vi "temp chart with pid.vi"(0 "Slave Controls":bool, 1 "exit T control":bool, 7 "Control Parameters":T4={"Setpoint"=50.0, "Control bandwidth"=4.0, "Settle bandwidth"=1.0, "Integral time"=30.0, "Int\non"=TRUE, "Derivative time"=0.5, "Der\non"=TRUE, "Settle time"=60.0} {"Settle time" format="%.2f"; "Derivative time" format="%.2f"; "Integral time" format="%.2f"; "Settle bandwidth" format="%.2f"; "Control bandwidth" format="%.2f"; "Setpoint" format="%.2f"}, 11 "error in":errorcluster, 12 "Manual Override":bool) -> (8 "Temp":dbl format="%.2f", 10 "Time in Settle Band":dbl format="%.2f", 14 "settled":bool, 15 "error out":errorcluster)   [LabVIEW 2016]
doc: "This vi records and plots the temperature of a 10 kOhm thermsitor using an Agilent 34405A as the measurment device.\n\nIt sets the power to the heater resistor using the NI ELVIS Variable DC, and measures the power using DAQ analog in.\n\nIt uses a PID feedback algorithm to obtain the desired setpoint.\n\nPaul K Dixon\nPhysics 350\nCSUSB Physics"
uses:
  typedefs/control parameters.ctl
  typedefs/status indicator.ctl
  typedefs/scale control.ctl
  <vilib>/Utility/miscctls.llb/LVPointTypeDef.ctl
  globals/temp control global variables.vi
panel:
  in  "Slave Scale":bool=TRUE
  out "Logging":bool
  in  "Scale Control":T1
  in  "Power Control":dbl(slide) scale=0.0..1.0
  out "range indicators":T2={"In control band"=FALSE, "In settle band"=FALSE, "under range"=TRUE, "over range"=FALSE}
  out "Power":dbl=0.754407202908737 format="%.2f"
  out "Setpoint":dbl=50.0 format="%.2f"
  in  "shrink":bool
  in  "expand":bool
  out "Temperature History":T3(graph)={"temp out"=29.702811899974034, 50.0, 50.5, 49.5, 50.1, 49.9, 50.508814405817475}
  # "PID Temperature Controller"
  # "1.0"
  # "Norm\nPower\nscale"
  # "0.5"
  # "0.0"
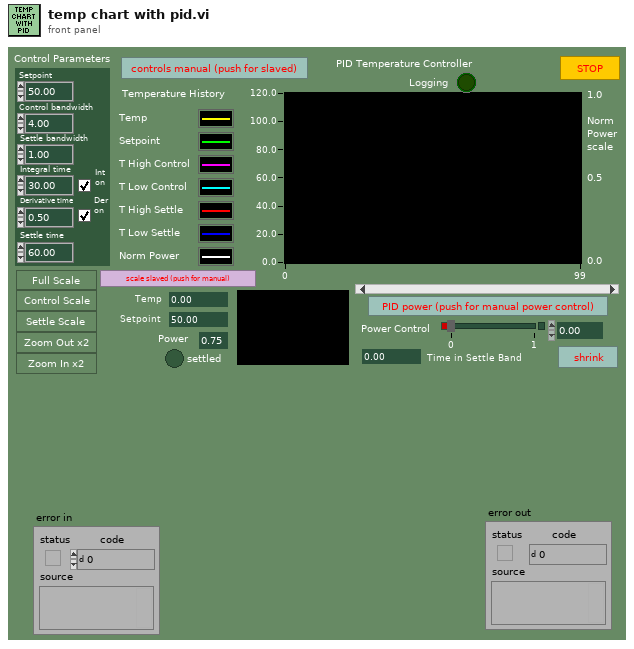
[diagram p1: front panel]
types:
  T1 = typedef "scale control.ctl" = cluster{"Full Scale":bool, "Control Scale":bool, "Settle Scale":bool, "Zoom Out":bool, "Zoom In":bool}
  T2 = typedef "status indicator.ctl" = cluster{"In control band":bool, "In settle band":bool, "under range":bool, "over range":bool}
  T3 = cluster{"temp out":dbl, dbl, dbl, dbl, dbl, dbl, dbl}
  T4 = typedef "control parameters.ctl" = cluster{"Setpoint":dbl, "Control bandwidth":dbl, "Settle bandwidth":dbl, "Integral time":dbl, "Int\non":bool, "Derivative time":dbl, "Der\non":bool, "Settle time":dbl}
  T5 = typedef "LVPointTypeDef.ctl" = cluster{"Horizontal":i16, "Vertical":i16}
  T6 = cluster{"[0]":refnum<vi>, "[1]":refnum<vi>, "[2]":refnum<vi>, "[3]":refnum<vi>}
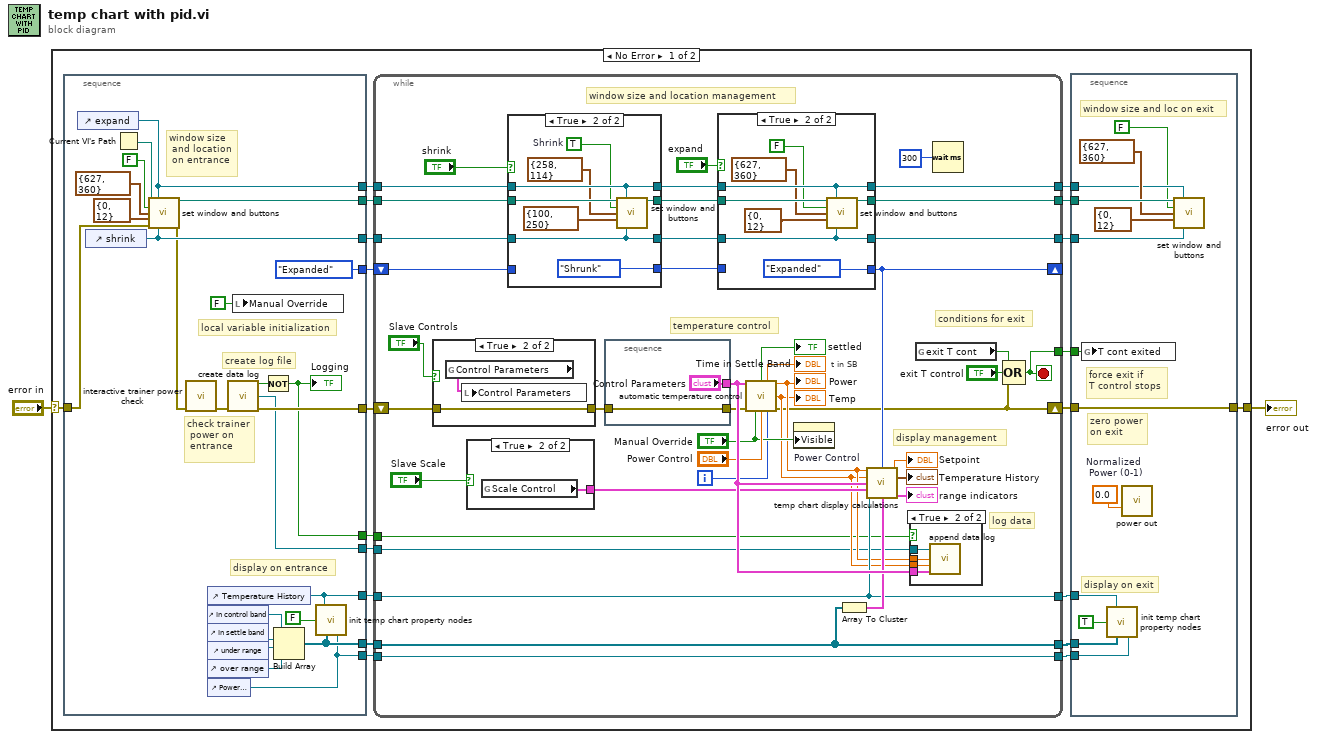
[diagram p0: block diagram]
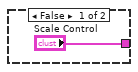
[diagram p2: hidden frame]
diagram:
  n1 = case shown="No Error" "error in" {
    selector: "error in" -> [w20 w137]
    tunnel: [w21 w137] -> w1
    frame No Error {
      n2 = stacked-sequence {
        tunnel: w20 -> [w128]
        tunnel: [w135] -> w19
        tunnel: [w130] -> w17
        tunnel: [w129] -> w16
        tunnel: [w125] -> w12
        tunnel: [w126] -> w11
        tunnel: [w123] -> w7
        tunnel: [w121] -> w6
        tunnel: [w118] -> w5
        tunnel: [w117] -> w4
        tunnel: [enum16{"Expanded", "Shrunk"}."Expanded" ("Mode")] -> w3
        frame #0 {
          # "create log file"
          # "local variable initialization"
          # "display on entrance"
          # "check trainer\n power on\n entrance"
          # "window size\n and location\n on entrance"
          n3 = control-ref of="expand"() -> (w130:refnum<vi>)
          n4 = control-ref of="shrink"() -> (w129:refnum<vi>)
          n5 = Current VI's Path() -> (path=w136:path)
          n6 = call "set window and buttons.vi"("path in"=w136, "expand ref"=w130, "Shrink"=FALSE, "Window Dimensions"=cluster{"window width":i16, "window height":i16} {"window width"=627, "window height"=360} ("Default LTWH"), "Origin"=T5 {"Horizontal"=0, "Vertical"=12}, "error in"=w128, "shrink ref"=w129) -> ("path out"=w135:path, "error out"=w127:errorcluster)  [unwired: 7 out]
          n7 = call "interactive trainer power check.vi"("error in"=w127) -> ("error out"=w122:errorcluster)  [unwired: 14 out]
          n8 = control-ref of="Temperature History"() -> (w126:refnum<vi>)
          n9 = control-ref of="In control band"() -> (w131:refnum<vi>)
          n10 = control-ref of="In settle band"() -> (w132:refnum<vi>)
          n11 = control-ref of="under range"() -> (w133:refnum<vi>)
          n12 = control-ref of="over range"() -> (w134:refnum<vi>)
          n13 = control-ref of="Power Control"() -> (w123:refnum<vi>)
          n14 = call "create data log.vi"("error in"=w122) -> ("cancelled"=w119:bool, "file refnum out"=w118:refnum<file>, "error out"=w121:errorcluster)  [unwired: 1 in, 11 out]
          n15 = local write "Manual Override"(FALSE ("Manual Override")) -> ()
          n16 = Not(x=w119) -> (.not. x?=w117:bool)
          "Logging" <- w117
          n17 = Build Array(w131, w132, w133, w134) -> (w125:refnum<vi>[])
          n18 = call "init temp chart property nodes.vi"("Temperature History"=w126, "Power control visible"=FALSE ("Visible"), "range indicators"=w125, "Power Control"=w123) -> ()  [unwired: 2 in, 10 out]
        }
      }
      n19 = while {
        tunnel: w7 -> [w37]
        tunnel: [w37] -> w8
        tunnel: [w38] -> w9
        tunnel: [w39] -> w10
        tunnel: w11 -> [w38]
        tunnel: w12 -> [w39]
        tunnel: [w41] -> w13
        tunnel: [w42] -> w14
        tunnel: [w43] -> w15
        tunnel: w16 -> [w48]
        tunnel: w17 -> [w49]
        tunnel: [w51] -> w18
        tunnel: w19 -> [w62]
        shift-left: w6 -> [w26]
        shift-right: [w27] -> w22
        tunnel: w5 -> [w32]
        tunnel: w4 -> [w31]
        shift-right: [w28] -> _
        shift-left: w3 -> [w30]
        i -> [w35]
        stop <- w51 stop-if-true
        # "log data"
        # "display management"
        # "conditions for exit"
        # "temperature control"
        # "t in SB"
        # "window size and location management"
        n20 = case shown="True" "Slave Controls" {
          tunnel: w26 -> [w67 w68]
          tunnel: [w67 w68] -> w25
          frame False {
          }
          frame True {
            n21 = global read "temp control global variables.vi" "Control Parameters"() -> (w69:T4)
            n22 = local write "Control Parameters"(w69) -> ()
          }
        }
        n23 = case shown="True" "Slave Scale" {
          tunnel: ["Scale Control" w66] -> w53
          frame False {
          }
          frame True {
            n24 = global read "temp control global variables.vi" "Scale Control"() -> (w66:T1)
          }
        }
        n25 = case shown="True" "shrink" {
          tunnel: w62 -> [w91 w99]
          tunnel: [w91 w98] -> w46
          tunnel: w49 -> [w90 w97]
          tunnel: w48 -> [w89 w96]
          tunnel: [w90 w97] -> w45
          tunnel: [w89 w96] -> w44
          tunnel: w30 -> [w88 _]
          tunnel: [w88 enum16{"Expanded", "Shrunk"}."Shrunk" ("Mode")] -> w29
          frame False {
          }
          frame True {
            w94 = TRUE  # Shrink
            n26 = call "set window and buttons.vi"("path in"=w99, "expand ref"=w97, "Shrink"=w94, "Window Dimensions"=cluster{"window width":i16, "window height":i16} {"window width"=258, "window height"=114} ("Default LTWH"), "Origin"=T5 {"Horizontal"=100, "Vertical"=250}, "shrink ref"=w96) -> ("path out"=w98:path)  [unwired: 1 in, 8 out]
          }
        }
        n27 = stacked-sequence {
          tunnel: ["Control Parameters"] -> w64
          tunnel: w25 -> [w86]
          tunnel: [w86] -> w50
          frame #0 {
          }
        }
        n28 = case shown="True" "expand" {
          tunnel: w46 -> [w77 w85]
          tunnel: [w77 w84] -> w43
          tunnel: w45 -> [w76 w83]
          tunnel: w44 -> [w75 w82]
          tunnel: [w76 w83] -> w41
          tunnel: [w75 w82] -> w42
          tunnel: w29 -> [w74 _]
          tunnel: [w74 enum16{"Expanded", "Shrunk"}."Expanded" ("Mode")] -> w28
          frame False {
          }
          frame True {
            n29 = call "set window and buttons.vi"("path in"=w85, "expand ref"=w83, "Shrink"=FALSE, "Window Dimensions"=cluster{"window width":i16, "window height":i16} {"window width"=627, "window height"=360} ("Default LTWH"), "Origin"=T5 {"Horizontal"=0, "Vertical"=12}, "shrink ref"=w82) -> ("path out"=w84:path)  [unwired: 1 in, 8 out]
          }
        }
        n30 = call "automatic temperature control.vi"("Control Parameters"=w64, "error in"=w50, "Manual Override"="Manual Override", "Normalized Power In (0-1)"="Power Control", "index (0=init)"=w35) -> ("settled"=→"settled":bool, "time in settle band"=→"Time in Settle Band":dbl, "power meas (0-1)"=w34:dbl, "temp meas"=w33:dbl, "error out"=w27:errorcluster)  [unwired: 2 in, 4 out]
        "Temp" <- w33
        "Power" <- w34
        n31 = property on="Power Control" class="Slide (strict)"("Visible"="Manual Override") -> ()  [unwired: 2 in, 2 out]
        n32 = Array To Cluster(array=w39) -> (cluster=w40:T6)
        n33 = call "temp chart display calculations.vi"("power in (0-1)"=w34, "Mode"=w28, "temp in"=w33, "Control Parameters"=w64, "Scale Control In"=w53, "Temp History in"=w38, "range indicator refs"=w40) -> ("Setpoint out"=→"Setpoint":dbl, "Temperature History out"=→"Temperature History":T3, "range indicators out"=→"range indicators":T2)  [unwired: 2 in, 4 out]
        n34 = case shown="True" w31 {
          tunnel: w34 -> [_ w73]
          tunnel: w33 -> [_ w72]
          tunnel: w64 -> [_ w71]
          tunnel: w32 -> [_ w70]
          frame False {
          }
          frame True {
            n35 = call "append data log.vi"("file refnum in"=w70, "Power"=w73, "Temp"=w72, "Control Parameters"=w71) -> ()  [unwired: 12 out]
          }
        }
        n36 = global read "temp control global variables.vi" "exit T cont"() -> (w36:bool)
        n37 = Wait (ms)(milliseconds to wait=u32 300) -> ()  [unwired: 1 out]
        n38 = Compound Arithmetic op=OR(w36, "exit T control", w27) -> (w51:bool)
      }
      n39 = stacked-sequence {
        tunnel: [w112] -> w21
        tunnel: w22 -> [w112]
        tunnel: w18 -> [w104]
        tunnel: w15 -> [w110]
        tunnel: w14 -> [w109]
        tunnel: w13 -> [w102]
        tunnel: w10 -> [w108]
        tunnel: w8 -> [w106]
        tunnel: w9 -> [w105]
        frame #0 {
          w111 = 0.0  # Normalized  Power (0-1)
          # "display on exit"
          # "force exit if \nT control stops"
          # "zero power\non exit"
          # "window size and loc on exit"
          n40 = global write "temp control global variables.vi" "T cont exited"(w104) -> ()
          n41 = call "init temp chart property nodes.vi"("Temperature History"=w105, "Power control visible"=TRUE ("Visible"), "range indicators"=w108, "Power Control"=w106) -> ()  [unwired: 2 in, 10 out]
          n42 = call "power out.vi"("Normalized Power (0-1)"=w111) -> ()  [unwired: 2 in, 13 out]
          n43 = call "set window and buttons.vi"("path in"=w110, "expand ref"=w102, "Shrink"=FALSE, "Window Dimensions"=cluster{"window width":i16, "window height":i16} {"window width"=627, "window height"=360} ("Default LTWH"), "Origin"=T5 {"Horizontal"=0, "Vertical"=12}, "shrink ref"=w109) -> ()  [unwired: 1 in, 9 out]
        }
      }
    }
    frame Error {
    }
  }
  "error out" <- w1
